vi "UpdateDa.vi"(8 "error in (no error)":errorcluster, 10 "RAW":bool, 11 "Sig_DA in":refnum<class "DA.lvclass">) -> (0 "error out":errorcluster, 2 "CURR":bool, 3 "Sig_DA out":refnum<class "DA.lvclass">)   [LabVIEW 2019, in "DA.lvclass"]
uses:
  DA.lvclass
  D:/GIT H4000/H4000/src/Proccess_class/Proccess.lvclass
  DA.lvclass/DA.ctl
  Proccess_class/Proccess.lvclass/Proccess.ctl
  Proccess_class/GetNames.vi
  Proccess_class/GetLogger.vi
  Logger_class/WriteEvent.vi
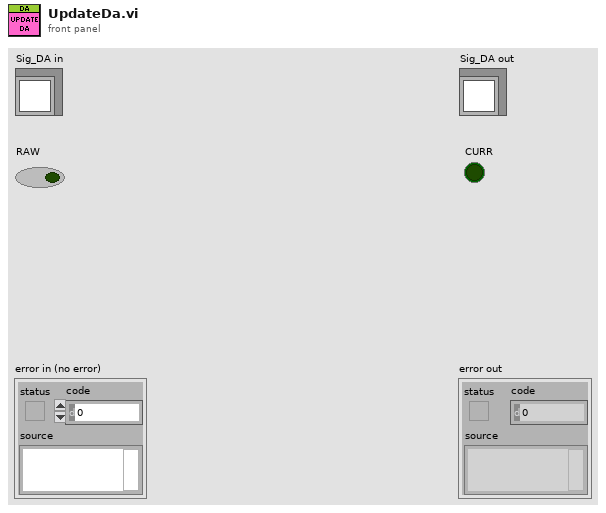
[diagram p1: front panel]
types:
  T1 = typedef "bool_data.ctl" = cluster{"CURR":bool, "RAW_PREV":bool, "millisecond timer value":u32}
  T2 = typedef "bool_setting.ctl" = cluster{"TON_ms":u32, "TOFF_ms":u32}
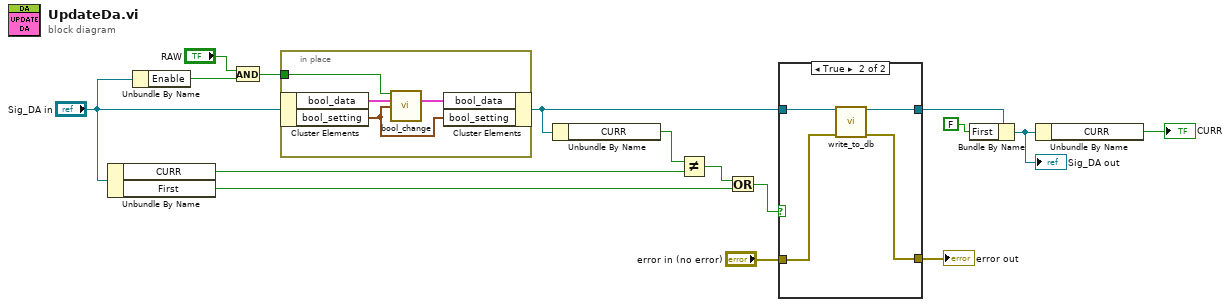
[diagram p0: block diagram]
diagram:
  n1 = Unbundle By Name("Sig_DA in") -> ("CURR"=w10:bool, "First"=w4:bool)
  n2 = Unbundle By Name("Sig_DA in") -> ("Enable"=w1:bool)
  n3 = And(x="RAW", y=w1) -> (x .and. y?=w2:bool)
  n4 = in-place {
    in-place-border: w2 -> [w17]
    n5 = in-place-cluster #1("Sig_DA in") -> ("bool_data"=w20:T1, "bool_setting"=w18:T2)
    n6 = call "bool_change.vi"("RAW"=w17, "bool_data_in"=w20, "bool_setting"=w18) -> ("bool_data_out"=w19:T1)  [unwired: 11 in, 1 out]
    n7 = in-place-cluster #1("bool_data"=w19, "bool_setting"=w18) -> (w8:refnum<class "DA.lvclass">)
  }
  n8 = Unbundle By Name(w8) -> ("CURR"=w9:bool)
  n9 = Not Equal?(x=w9, y=w10) -> (x != y?=w6:bool)
  n10 = Or(x=w6, y=w4) -> (x .or. y?=w5:bool)
  n11 = case shown="True" w5 {
    tunnel: w8 -> [w22 w26]
    tunnel: [w22 w25] -> w7
    tunnel: "error in (no error)" -> [w21 w24]
    tunnel: [w21 w23] -> w14
    frame False {
    }
    frame True {
      n12 = call "write_to_db.vi"("reference in"=w26, "error in (no error)"=w24) -> ("reference out"=w25:refnum<class "DA.lvclass">, "error out"=w23:errorcluster)  [unwired: 12 in]
    }
  }
  "error out" <- w14
  n13 = Bundle By Name(cluster=w7, "First"=FALSE) -> (w12:refnum<class "DA.lvclass">)
  "Sig_DA out" <- w12
  n14 = Unbundle By Name(w12) -> ("CURR"=→"CURR":bool)
